vi "Close_Baxter.vi"(0 "error in":errorcluster, 2 "topic":string, 3 "node":string) -> (1 "error out":errorcluster)   [LabVIEW 2012]
doc: "Closes a topic. If no topic is defined, it will close all topics and disable Baxter."
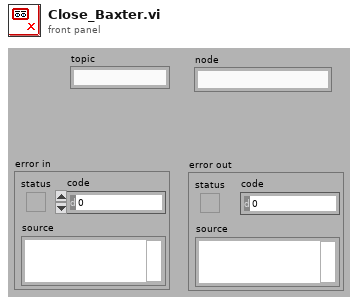
[diagram p1: front panel]
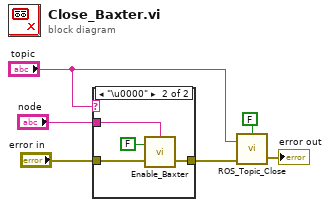
[diagram p0: block diagram]
diagram:
  n1 = case shown="\"\"" "topic" {
    tunnel: "error in" -> [w7 w11]
    tunnel: [w7 w10] -> w3
    tunnel: "node" -> [_ w8]
    frame Default {
    }
    frame "\u0000" {
      n2 = call <userlib>:"Enable_Baxter.vi"("error in"=w11, "Enable?"=FALSE, "node"=w8) -> ("error out"=w10:errorcluster)  [unwired: 1 in]
    }
  }
  n3 = call <userlib>:"ROS_Topic_Close.vi"("error in"=w3, "topic"="topic", "StopConsole"=FALSE) -> ("error out"=→"error out":errorcluster)  [unwired: 1 in]
